vi "CheckTemp.vi"(9 "MinTempLimit":dbl, 10 "NtcNumber":u64, 11 "Temp_In":dbl[](array[numeric])) -> (0 "error out":errorcluster, 2 "Report Text":string, 3 "Temp":dbl[](array[numeric]))   [LabVIEW 2013]
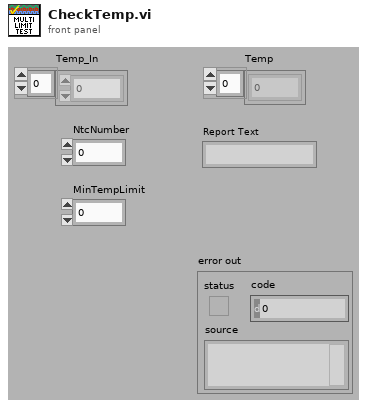
[diagram p1: front panel]
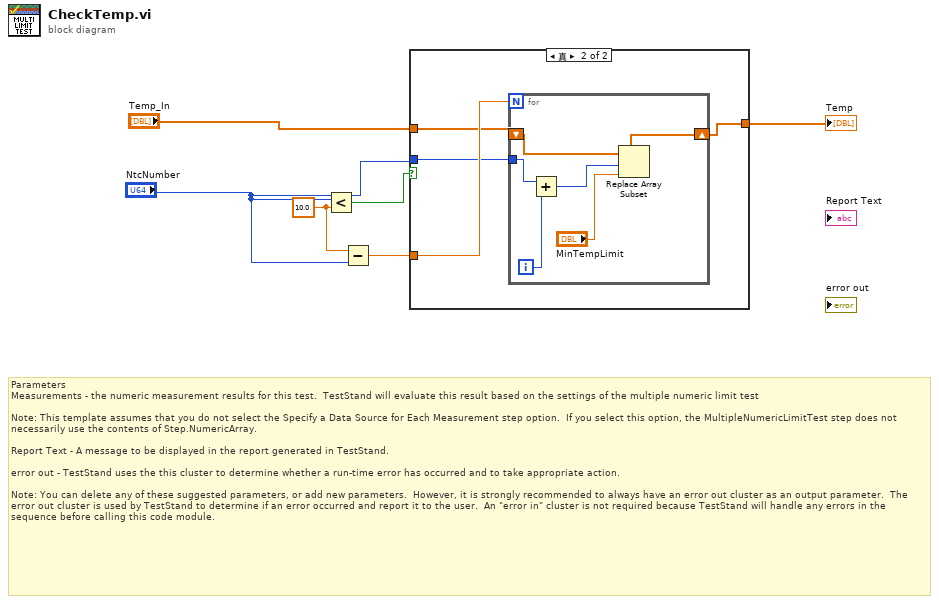
[diagram p0: block diagram]
diagram:
  w3 = 10.0 ("y")
  # "Parameters\nMeasurements - the numeric measurement results for this test.  TestStand will evaluate this result based on the settings of the multiple numeric limit test\n\nNote: This template assumes that you do not select the Specify a Data Source for Each Measurement step option.  If you select this option, the MultipleNumericLimitTest step does not necessarily use the contents of Step.NumericArray. \n\nReport Text - A message to be displayed in the report generated in TestStand. \n\nerror out - TestStand uses the this cluster to determine whether a run-time error has occurred and to take appropriate action.  \n\nNote: You can delete any of these suggested parameters, or add new parameters.  However, it is strongly recommended to always have an error out cluster as an output parameter.  The error out cluster is used by TestStand to determine if an error occurred and report it to the user.  An \"error in\" cluster is not required because TestStand will handle any errors in the sequence before calling this code module."
  n1 = Less?(x="NtcNumber", y=w3) -> (x < y?=w6:bool)
  n2 = Subtract(x=w3, y="NtcNumber") -> (x-y=w2:dbl)
  n3 = case shown="真" w6 {
    tunnel: "Temp_In" -> [w7 w10]
    tunnel: [w7 w8] -> w4
    tunnel: w2 -> [_ w11]
    tunnel: "NtcNumber" -> [_ w9]
    frame False {
    }
    frame True {
      n4 = for {
        N: w11 -> [_]
        shift-right: [w16] -> w8
        shift-left: w10 -> [w17]
        tunnel: w9 -> [w15]
        i -> [w14]
        n5 = Add(x=w15, y=w14) -> (x+y=w13:u64)
        n6 = Replace Array Subset(array=w17, new element="MinTempLimit", index=w13) -> (w16:dbl[])
      }
    }
  }
  "Temp" <- w4
